vi "Navigation encode.vi"(11 "Array":dbl[](array[numeric])=[111.12345886230469, 111.12345886230469, 111.12345886230469, 9199.099609375, 9299.2001953125, 9399.5, 9499.599609375, 9599.7001953125, 9699.7998046875, 9799.900390625] format="%#.8g") -> (3 "Navigation string":string)   [LabVIEW 2021]
panel:
  out "value 3":i16[](array[numeric])
  out "value 2":i8[](array[numeric])
  out "value":sgl[](array[numeric])
  out "length 4":i32
  out "length 3":i32
  out "length 2":i32
  out "length":i32
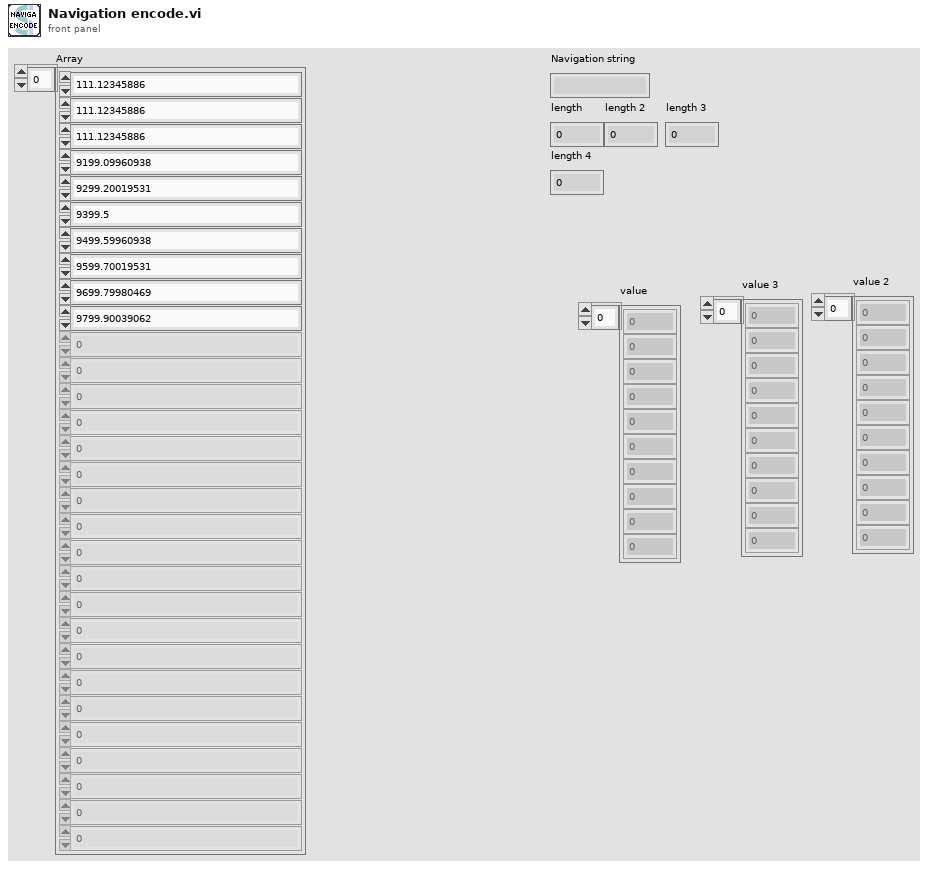
[diagram p1: front panel]
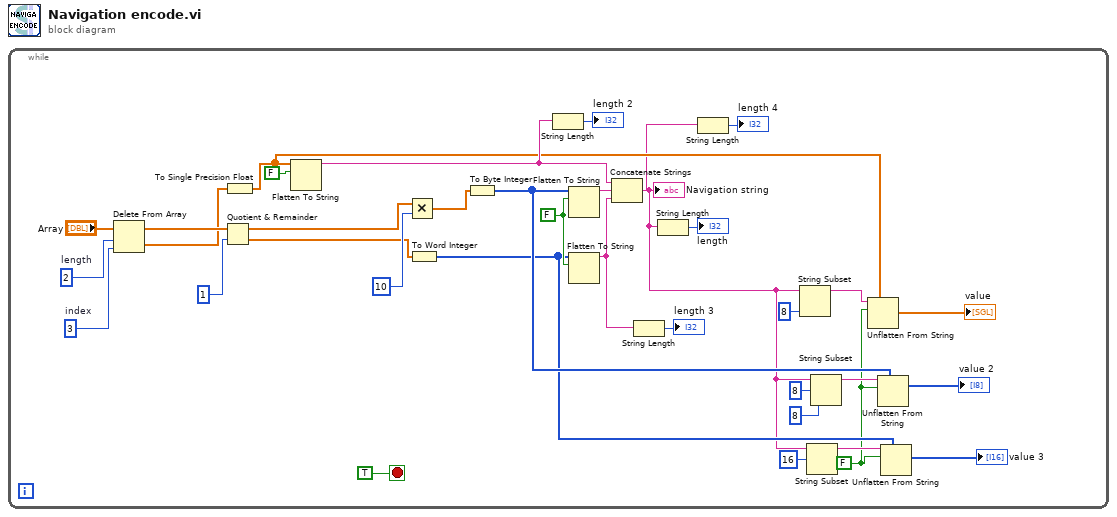
[diagram p0: block diagram]
diagram:
  n1 = while {
    stop <- TRUE stop-if-true
    w5 = FALSE ("data includes array or string size? (T)")
    w26 = FALSE ("prepend array or string size? (T)")
    w34 = 2  # length
    w35 = 3  # index
    n2 = Delete From Array "Delete From Array"(array="Array", length=w34, index=w35) -> (deleted portion=w25:dbl[], array with subset deleted=w27:dbl[])
    n3 = Quotient & Remainder(x=w27, y=1) -> (x-y*floor(x/y)=w32:dbl[], floor(x/y)=w29:dbl[])
    n4 = To Single Precision Float(number=w25) -> (single precision float=w17:sgl[])
    n5 = Flatten To String(anything=w17, prepend array or string size? (T)=FALSE) -> (data string=w20:string)  [unwired: 2 in, 2 out]
    n6 = Multiply(x=w32, y=10) -> (x*y=w30:dbl[])
    n7 = To Word Integer(number=w29) -> (16bit integer=w15:i16[])
    n8 = To Byte Integer(number=w30) -> (8bit integer=w16:i8[])
    n9 = String Length(string=w20) -> (length=→"length 2":i32)
    n10 = Flatten To String(anything=w16, prepend array or string size? (T)=w26) -> (data string=w3:string)  [unwired: 2 in, 2 out]
    n11 = Flatten To String(anything=w15, prepend array or string size? (T)=w26) -> (data string=w18:string)  [unwired: 2 in, 2 out]
    n12 = Concatenate Strings(w20, w3, w18) -> (w14:string)
    "Navigation string" <- w14
    n13 = String Length(string=w18) -> (length=→"length 3":i32)
    n14 = String Length(string=w14) -> (length=→"length":i32)
    n15 = String Length(string=w3) -> (length=→"length 4":i32)
    n16 = String Subset(string=w14, length (rest)=8 ("length (rest)")) -> (substring=w13:string)  [unwired: 1 in]
    n17 = String Subset(string=w14, offset (0)=16) -> (substring=w11:string)  [unwired: 1 in]
    n18 = String Subset(string=w14, offset (0)=8, length (rest)=8 ("length (rest)")) -> (substring=w12:string)
    n19 = Unflatten From String(type=w17, binary string=w13, data includes array or string size? (T)=w5) -> (value=→"value":sgl[])  [unwired: 2 in, 2 out]
    n20 = Unflatten From String(type=w16, binary string=w12, data includes array or string size? (T)=w5) -> (value=→"value 2":i8[])  [unwired: 2 in, 2 out]
    n21 = Unflatten From String(type=w15, binary string=w11, data includes array or string size? (T)=w5) -> (value=→"value 3":i16[])  [unwired: 2 in, 2 out]
  }
